vi "EFMC-2.vi"(11 "数组":u8[](array[numeric])) -> (1 "GLOADSST辅助数据有效字":T5, 2 "系统故障字1":T4, 3 "组合状态 字":T3, 4 "GPSBD辅助数据有效字":T6, 5 "组合模式受控状态":cluster{"自动":bool, " 强选":bool}, 6 "组合导航数据有效字":T1, 7 "惯组数据有效字":T2)   [LabVIEW 2012]
uses:
  index-i16.vi
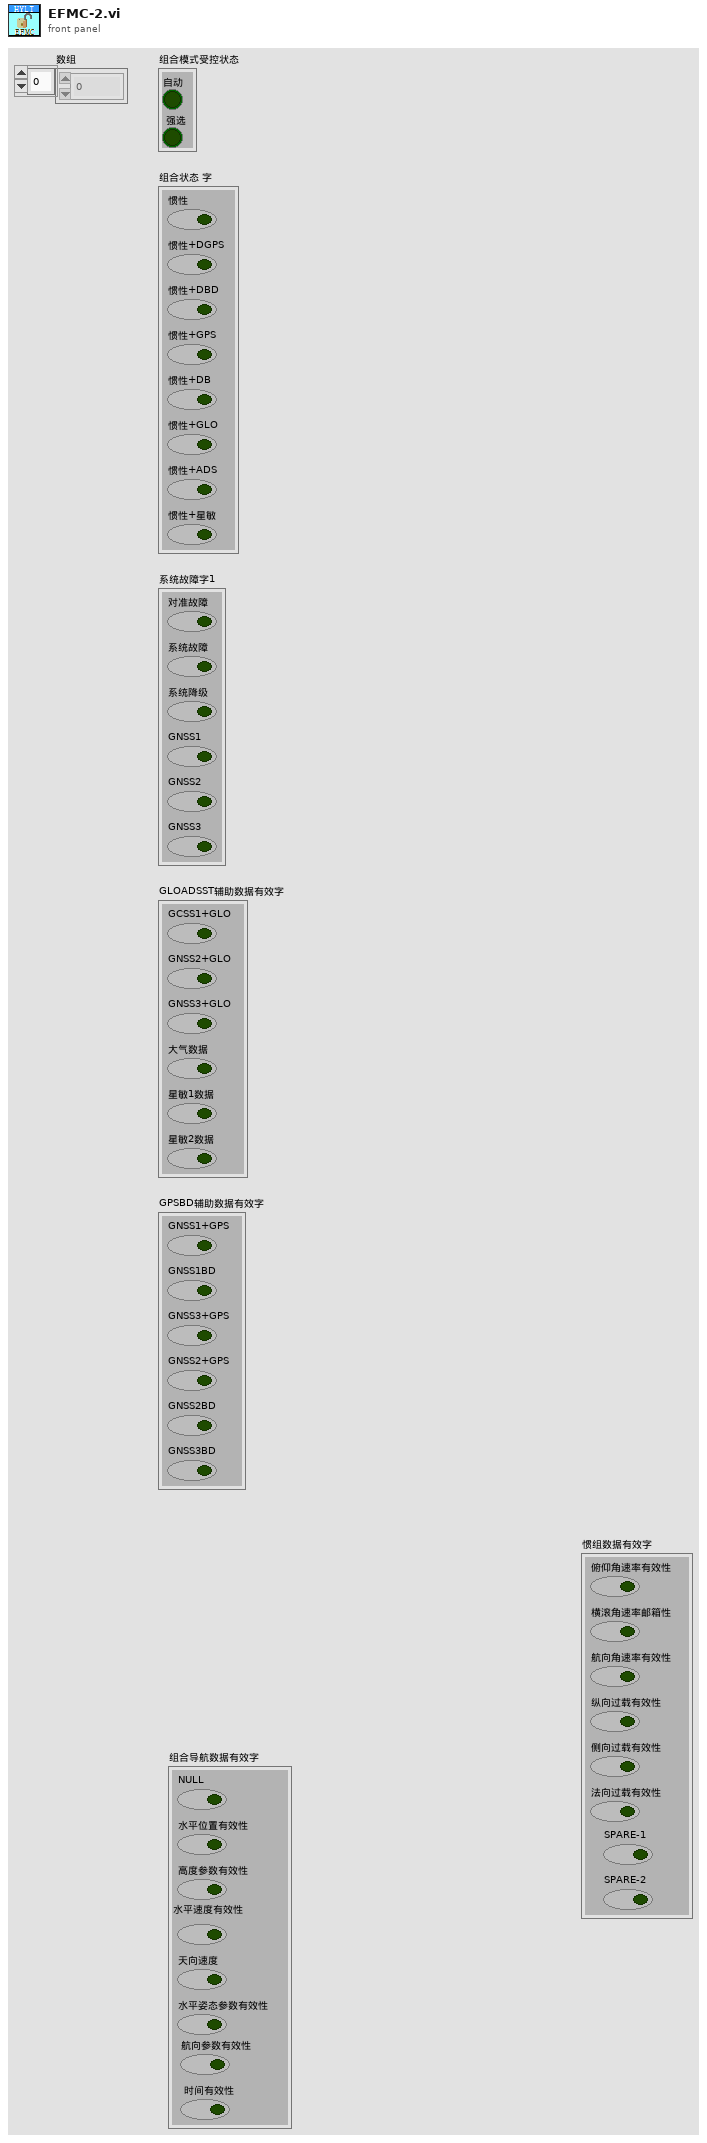
[diagram p1: front panel]
types:
  T1 = cluster{"NULL":bool, "水平位置有效性":bool, "高度参数有效性":bool, "水平速度有效性":bool, "天向速度":bool, "水平姿态参数有效性":bool, " 时间有效性":bool, "航向参数有效性":bool}
  T2 = cluster{"俯仰角速率有效性":bool, "横滚角速率邮箱性":bool, "航向角速率有效性":bool, "纵向过载有效性":bool, "侧向过载有效性":bool, "法向过载有效性":bool, "SPARE-2":bool, "SPARE-1":bool}
  T3 = cluster{"惯性":bool, "惯性+DGPS":bool, "惯性+DBD":bool, "惯性+GPS":bool, "惯性+DB":bool, "惯性+GLO":bool, "惯性+ADS":bool, "惯性+星敏":bool}
  T4 = cluster{"对准故障":bool, "系统故障":bool, "系统降级":bool, "GNSS1":bool, "GNSS2":bool, "GNSS3":bool}
  T5 = cluster{"GCSS1+GLO":bool, "GNSS2+GLO":bool, "GNSS3+GLO":bool, "大气数据":bool, "星敏1数据":bool, "星敏2数据":bool}
  T6 = cluster{"GNSS1+GPS":bool, "GNSS1BD":bool, "GNSS3+GPS":bool, "GNSS2+GPS":bool, "GNSS2BD":bool, "GNSS3BD":bool}
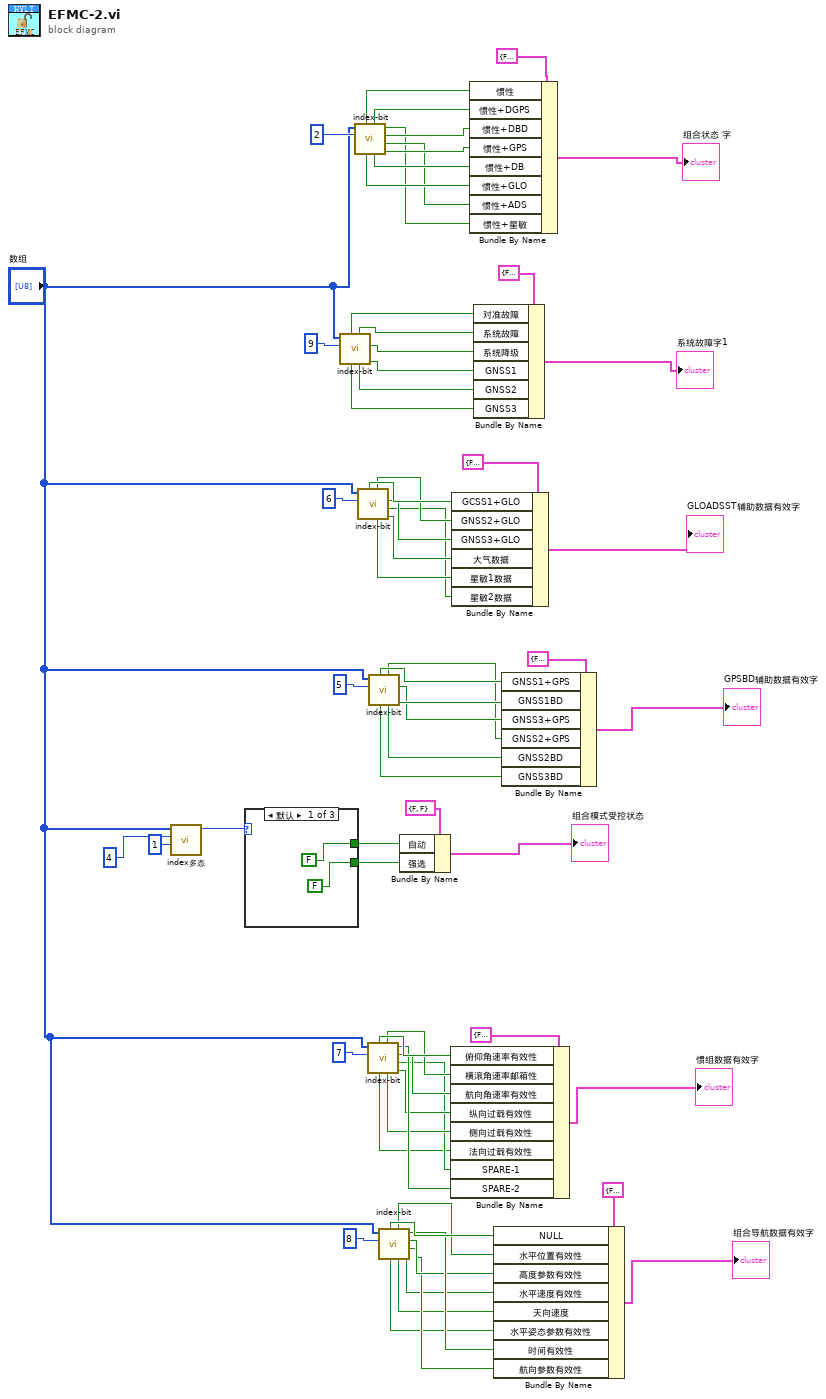
[diagram p0: block diagram]
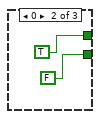
[diagram p2: hidden frame]
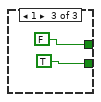
[diagram p3: hidden frame]
diagram:
  n1 = call-poly "index多态.vi"("长度"=1, "索引"=4, "数组"="数组") -> ("数值输出"=w66:i16)  [unwired: 8 in]
  n2 = case shown="默认" w66 {
    tunnel: [FALSE TRUE FALSE] -> w67
    tunnel: [FALSE FALSE TRUE] -> w68
    frame Default {
    }
    frame 0 {
    }
    frame 1 {
    }
  }
  n3 = call "index-bit.vi"("index"=9 ("索引"), "array"="数组") -> ("bit3"=w47:bool, "bit2"=w48:bool, "bit4"=w46:bool, "bit1"=w49:bool, "bit5"=w45:bool, "bit0"=w50:bool)  [unwired: 2 in, 2 out]
  n4 = call "index-bit.vi"("index"=2 ("索引"), "array"="数组") -> ("bit3"=w56:bool, "bit6"=w53:bool, "bit2"=w57:bool, "bit7"=w52:bool, "bit4"=w55:bool, "bit1"=w58:bool, "bit5"=w54:bool, "bit0"=w59:bool)  [unwired: 2 in]
  n5 = call "index-bit.vi"("index"=6 ("索引"), "array"="数组") -> ("bit3"=w35:bool, "bit6"=w33:bool, "bit2"=w36:bool, "bit4"=w34:bool, "bit1"=w37:bool, "bit0"=w38:bool)  [unwired: 2 in, 2 out]
  n6 = call "index-bit.vi"("index"=7 ("索引"), "array"="数组") -> ("bit3"=w12:bool, "bit6"=w10:bool, "bit2"=w13:bool, "bit7"=w14:bool, "bit4"=w11:bool, "bit1"=w15:bool, "bit5"=w9:bool, "bit0"=w16:bool)  [unwired: 2 in]
  n7 = call "index-bit.vi"("index"=5 ("索引"), "array"="数组") -> ("bit3"=w28:bool, "bit2"=w27:bool, "bit4"=w25:bool, "bit1"=w26:bool, "bit5"=w24:bool, "bit0"=w29:bool)  [unwired: 2 in, 2 out]
  n8 = call "index-bit.vi"("index"=8 ("索引"), "array"="数组") -> ("bit3"=w3:bool, "bit6"=w4:bool, "bit2"=w5:bool, "bit7"=w6:bool, "bit4"=w2:bool, "bit1"=w7:bool, "bit5"=w1:bool, "bit0"=w8:bool)  [unwired: 2 in]
  n9 = Bundle By Name(cluster=cluster{"自动":bool, " 强选":bool} {"自动"=FALSE, " 强选"=FALSE} ("组合模式受控状态"), "自动"=w67, "强选"=w68) -> (→"组合模式受控状态":cluster{"自动":bool, " 强选":bool})
  n10 = Bundle By Name(cluster=T2 {"俯仰角速率有效性"=FALSE, "横滚角速率邮箱性"=FALSE, "航向角速率有效性"=FALSE, "纵向过载有效性"=FALSE, "侧向过载有效性"=FALSE, "法向过载有效性"=FALSE, "SPARE-2"=FALSE, "SPARE-1"=FALSE} ("惯组数据有效字"), "俯仰角速率有效性"=w16, "横滚角速率邮箱性"=w15, "航向角速率有效性"=w13, "纵向过载有效性"=w12, "侧向过载有效性"=w11, "法向过载有效性"=w9, "SPARE-1"=w10, "SPARE-2"=w14) -> (→"惯组数据有效字":T2)
  n11 = Bundle By Name(cluster=T5 {"GCSS1+GLO"=FALSE, "GNSS2+GLO"=FALSE, "GNSS3+GLO"=FALSE, "大气数据"=FALSE, "星敏1数据"=FALSE, "星敏2数据"=FALSE} ("GLOADSST辅助数据有效字"), "GCSS1+GLO"=w38, "GNSS2+GLO"=w37, "GNSS3+GLO"=w36, "大气数据"=w35, "星敏1数据"=w34, "星敏2数据"=w33) -> (→"GLOADSST辅助数据有效字":T5)
  n12 = Bundle By Name(cluster=T3 {"惯性"=FALSE, "惯性+DGPS"=FALSE, "惯性+DBD"=FALSE, "惯性+GPS"=FALSE, "惯性+DB"=FALSE, "惯性+GLO"=FALSE, "惯性+ADS"=FALSE, "惯性+星敏"=FALSE} ("组合状态"), "惯性"=w59, "惯性+DGPS"=w58, "惯性+DBD"=w57, "惯性+GPS"=w56, "惯性+DB"=w55, "惯性+GLO"=w54, "惯性+ADS"=w53, "惯性+星敏"=w52) -> (→"组合状态 字":T3)
  n13 = Bundle By Name(cluster=T4 {"对准故障"=FALSE, "系统故障"=FALSE, "系统降级"=FALSE, "GNSS1"=FALSE, "GNSS2"=FALSE, "GNSS3"=FALSE} ("系统故障"), "对准故障"=w50, "系统故障"=w49, "系统降级"=w48, "GNSS1"=w47, "GNSS2"=w46, "GNSS3"=w45) -> (→"系统故障字1":T4)
  n14 = Bundle By Name(cluster=T1 {"NULL"=FALSE, "水平位置有效性"=FALSE, "高度参数有效性"=FALSE, "水平速度有效性"=FALSE, "天向速度"=FALSE, "水平姿态参数有效性"=FALSE, " 时间有效性"=FALSE, "航向参数有效性"=FALSE} ("组合导航数据有效字"), "NULL"=w8, "水平位置有效性"=w7, "高度参数有效性"=w5, "水平速度有效性"=w3, "天向速度"=w2, "水平姿态参数有效性"=w1, "时间有效性"=w6, "航向参数有效性"=w4) -> (→"组合导航数据有效字":T1)
  n15 = Bundle By Name(cluster=T6 {"GNSS1+GPS"=FALSE, "GNSS1BD"=FALSE, "GNSS3+GPS"=FALSE, "GNSS2+GPS"=FALSE, "GNSS2BD"=FALSE, "GNSS3BD"=FALSE} ("GPSBD辅助数据有效字"), "GNSS1+GPS"=w29, "GNSS1BD"=w28, "GNSS3+GPS"=w27, "GNSS2+GPS"=w26, "GNSS2BD"=w25, "GNSS3BD"=w24) -> (→"GPSBD辅助数据有效字":T6)
